vi "add status update message to log.vi"(7 "Server Alias":string, 8 "Error In":errorcluster, 11 "Tcp Message":T1={"Command"="", "Data"=[], "Script ID"=0, "LabVIEW Server ID"="zxcvbnm,", "Python Message ID"=0}) -> (0 "Error Out":errorcluster)   [LabVIEW 2013, in "TS.lvlib"]
doc: "This VI addes the Data piece of the input to the Status global variable, as well as a timestamp to the Status TS array."
uses:
  TS.lvlib
  Status Message.ctl
  LabVIEW Python Connector Message.ctl
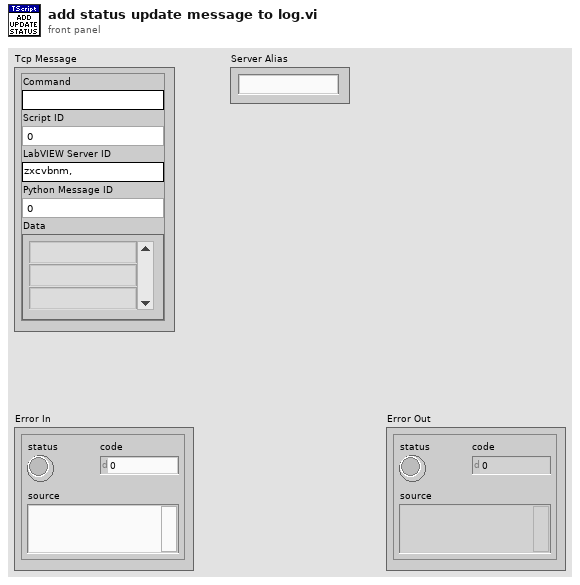
[diagram p1: front panel]
types:
  T1 = typedef "TS.lvlib/LabVIEW Python Connector Message.ctl" = cluster{"Command":string, "Data":string[], "Script ID":i64, "LabVIEW Server ID":string, "Python Message ID":i32}
  T2 = typedef "TS.lvlib/Status Message.ctl" = cluster{"Text":string, "Time":timestamp}
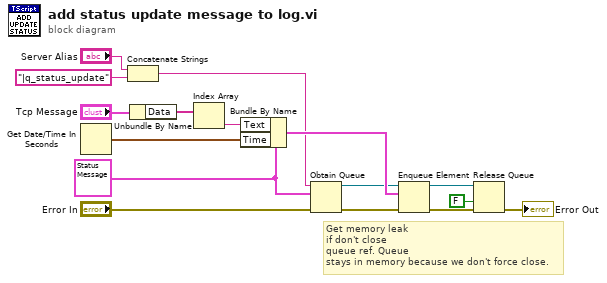
[diagram p0: block diagram]
diagram:
  w10 = T2 {"Text"="", "Time"=timestamp(0 s since 1904-01-01)} ("Status Update Message")
  # "Get memory leak\nif don't close \nqueue ref. Queue\nstays in memory because we don't force close."
  n1 = Get Date/Time In Seconds() -> (seconds since 1Jan1904=w13:timestamp)
  n2 = Concatenate Strings("Server Alias", "|q_status_update" ("name (unnamed)")) -> (w2:string)
  n3 = Unbundle By Name("Tcp Message") -> ("Data"=w15:string[])
  n4 = Index Array(array=w15) -> (element=w14:string)  [unwired: 1 in]
  n5 = Bundle By Name(cluster=w10, "Text"=w14, "Time"=w13) -> (w9:T2)
  n6 = Obtain Queue(name (unnamed)=w2, element data type=w10, error in (no error)="Error In") -> (queue out=w6:refnum<queue>, error out=w8:errorcluster)  [unwired: 2 in, 1 out]
  n7 = Enqueue Element(queue=w6, element=w9, error in (no error)=w8) -> (queue out=w4:refnum<queue>, error out=w5:errorcluster)  [unwired: 1 in, 1 out]
  n8 = Release Queue(queue=w4, force destroy? (F)=FALSE, error in (no error)=w5) -> (error out=→"Error Out":errorcluster)  [unwired: 2 out]
